vi "Teleop.vi"(10 "Match Info":T1={"Autonomous Elapsed Seconds"=0.0, "TeleOp Elapsed Seconds"=0.0, "Disabled Elapsed Seconds"=0.0, "Visited Autonomous"=FALSE, "Visited TeleOp"=FALSE, "Visited Disabled"=FALSE, "Autonomous Settings"={"Autonomous Style"=enum."Independent", "VI Refnum"=refnum}}, 11 "Call Context":T2) -> ()   [LabVIEW 2015]
doc: "This VI is called for each TeleOp packet received from the DS where the robot is not disabled. It is often used to read from the joysticks and update I/O or to update setpoints for timed control loops. It should complete and return within 20 milliseconds or it may miss DS packets."
uses:
  <vilib>/Rock Robotics/WPI/DriverStation/WPI_DriverStationDerivedRobotMode.ctl
  <vilib>/Rock Robotics/WPI/DriverStation/WPI_DriverStationMatch Info.ctl
  <vilib>/Rock Robotics/WPI/Utilities/WPI_GetSetVariantRefNum.vi
  <vilib>/Rock Robotics/Network Tables/NT Write Boolean Array.vi
  <vilib>/Rock Robotics/Network Tables/NT Write Numeric Array.vi
  <vilib>/Rock Robotics/Network Tables/NT Read Boolean.vi
  <vilib>/Rock Robotics/Network Tables/NT Read Number.vi
  Robot Global Data.vi
  <vilib>/Rock Robotics/Network Tables/NT Write Boolean.vi
panel:
  out "Sample Slider 0":dbl(slide) scale=0.0..5.0
  out "Sample Boolean 1":bool
  out "Sample Boolean 0":bool
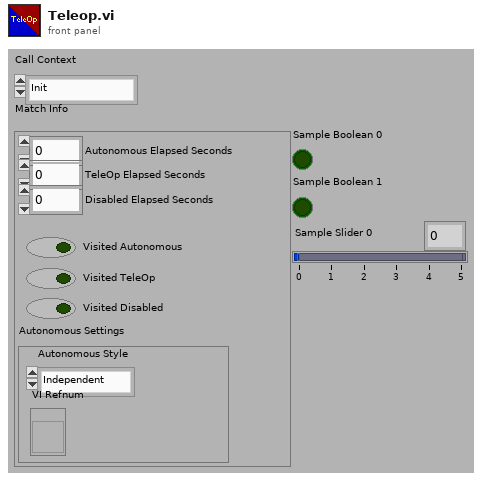
[diagram p1: front panel]
types:
  T1 = typedef "WPI_DriverStationMatch Info.ctl" = cluster{"Autonomous Elapsed Seconds":dbl, "TeleOp Elapsed Seconds":dbl, "Disabled Elapsed Seconds":dbl, "Visited Autonomous":bool, "Visited TeleOp":bool, "Visited Disabled":bool, "Autonomous Settings":cluster{"Autonomous Style":enum16{"Iterative", "Independent"}, "VI Refnum":refnum<vi>}}
  T2 = typedef "WPI_DriverStationDerivedRobotMode.ctl" = enum16{"Init", "Execute", "Stop"}
  T3 = typedef "WPI_RobotDriveDevRef.ctl" = cluster{"DevStatus":errorcluster, "Motors[]":T4[], "Square Inputs":bool, "Max Output":dbl}
  T4 = typedef "WPI_MotorControlDeviceRef.ctl" = cluster{"DeviceStatus":errorcluster, "Type":T5, "PWM":cluster{"PWM Channel":T6, "DeadBand":T7}, "CAN":cluster{"Device Number":u8, "Control Mode":T8, "Semaphore":T9, "Max Vout":dbl, "TalonSRX Control Mode":T10}, "Invert":bool}
  T5 = typedef "WPI_MotorControlType.ctl" = enum16{"PWM", "CAN", "CANTalonSRX"}
  T6 = typedef "FPGA_DIOPWMChannel.ctl" = enum8{"PWM 0", "PWM 1", "PWM 2", "PWM 3", "PWM 4", "PWM 5", "PWM 6", "PWM 7", "PWM 8", "PWM 9", "PWM MXP 0", "PWM MXP 1", "PWM MXP 2", "PWM MXP 3", "PWM MXP 4", "PWM MXP 5", "PWM MXP 6", "PWM MXP 7", "PWM MXP 8", "PWM MXP 9", "Invalid"}
  T7 = typedef "WPI_PWMDeadband.ctl" = cluster{"Name":string, "maxPositivePwm":i32, "minPositivePwm":i32, "centerPwm":i32, "maxNegativePwm":i32, "minNegativePwm":i32, "angularRange":u16}
  T8 = typedef "WPI_CANJaguar_ControlMode.ctl" = enum8{"Percent VBus", "Current", "Speed", "Position", "Voltage"}
  T9 = typedef "Semaphore RefNum" = refnum<k1>
  T10 = typedef "WPI_CANTalonSRX_APIControlMode.ctl" = enum8{"Percent VBus", "Speed", "Position", "Slave", "Unchanged / Invalid", "Voltage Compensation", "Current", "Motion Profile"}
  T11 = typedef "WPI_JoystickDevRef.ctl" = cluster{"Device":T12}
  T12 = typedef "WPI_JoystickDeviceEnum.ctl" = enum16{"USB 0", "USB 1", "USB 2", "USB 3", "USB 4", "USB 5"}
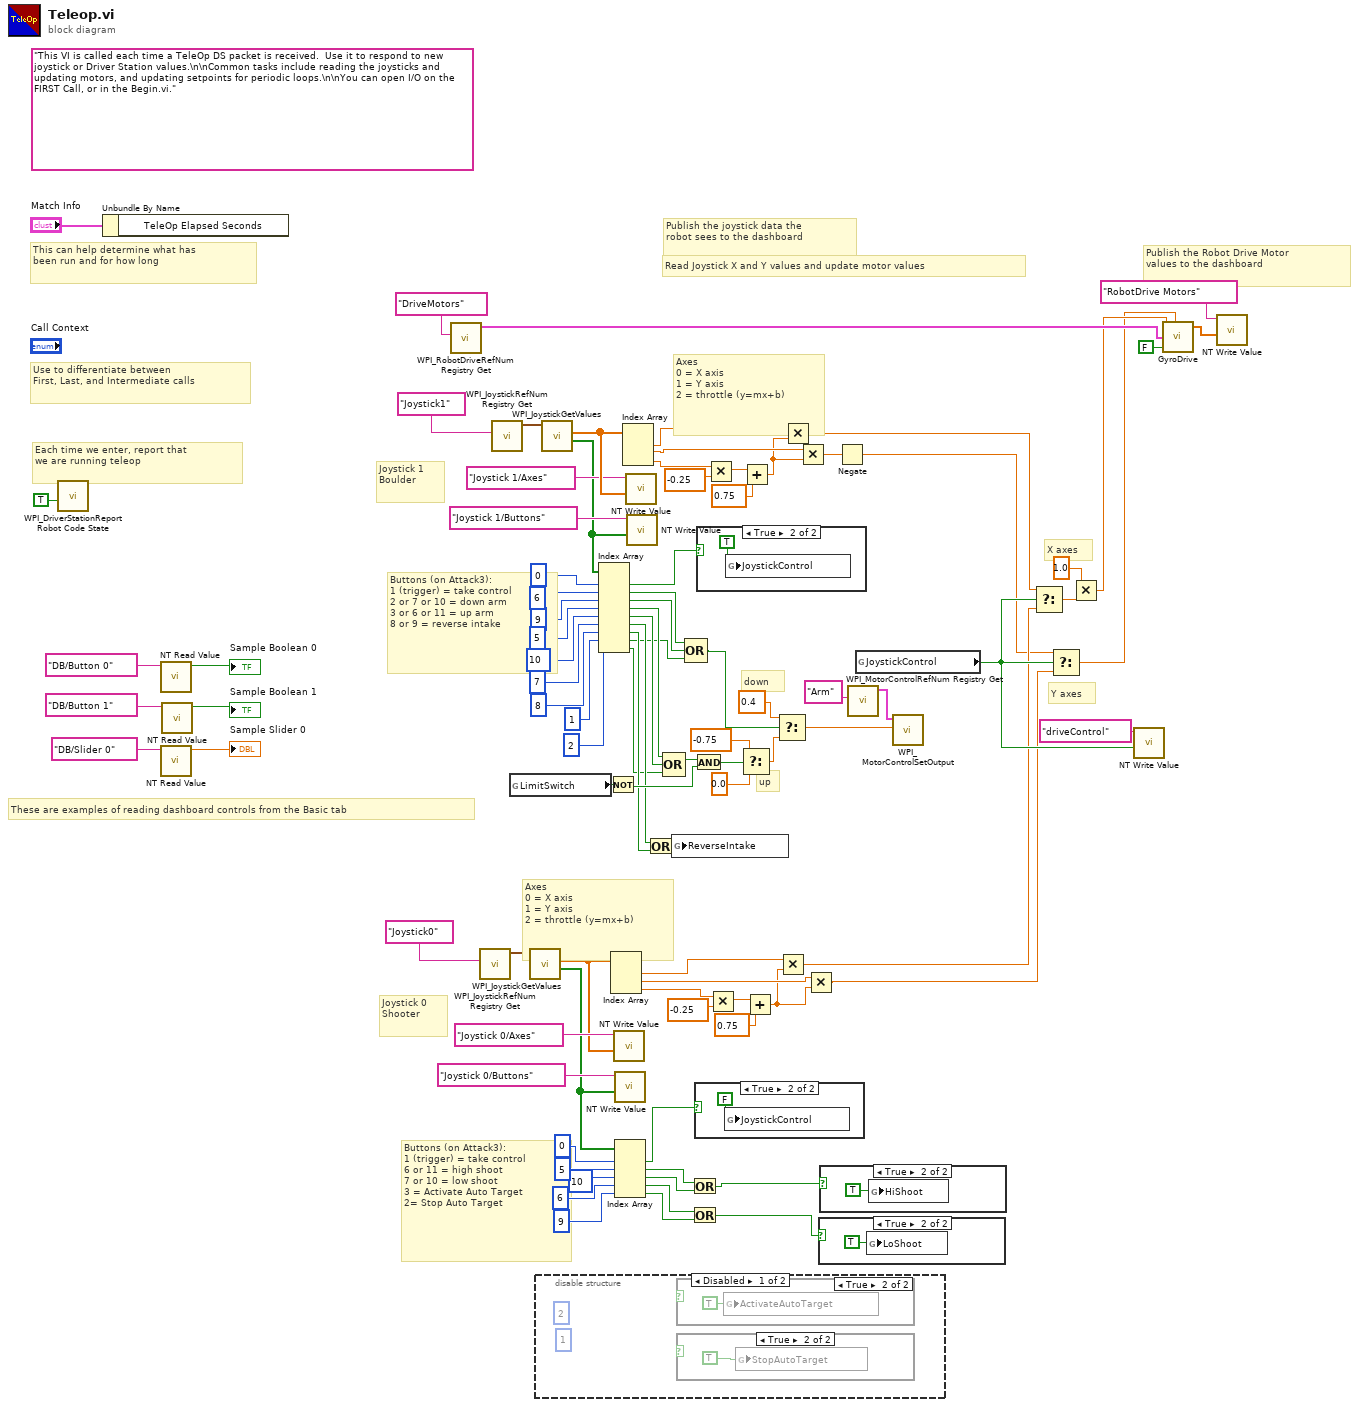
[diagram p0: block diagram]
diagram:
  (unwired) "This VI is called each time a TeleOp DS packet is received.  Use it to respond to new joystick or Driver Station values.\n\nCommon tasks include reading the joysticks and updating motors, and updating setpoints for periodic loops.\n\nYou can open I/O on the FIRST Call, or in the Begin.vi."
  # "up"
  # "down"
  # "Buttons (on Attack3):\n1 (trigger) = take control\n6 or 11 = high shoot\n7 or 10 = low shoot\n3 = Activate Auto Target\n2= Stop Auto Target"
  # "Buttons (on Attack3):\n1 (trigger) = take control\n2 or 7 or 10 = down arm\n3 or 6 or 11 = up arm\n8 or 9 = reverse intake"
  # "Axes\n0 = X axis\n1 = Y axis\n2 = throttle (y=mx+b)"
  # "Axes\n0 = X axis\n1 = Y axis\n2 = throttle (y=mx+b)"
  # "Y axes"
  # "X axes"
  # "Joystick 1\nBoulder"
  # "Joystick 0\nShooter"
  # "These are examples of reading dashboard controls from the Basic tab"
  # "Publish the Robot Drive Motor\nvalues to the dashboard"
  # "Publish the joystick data the\nrobot sees to the dashboard"
  # "Each time we enter, report that\nwe are running teleop"
  # "Use to differentiate between\nFirst, Last, and Intermediate calls"
  # "This can help determine what has\nbeen run and for how long"
  # "Read Joystick X and Y values and update motor values"
  n1 = call <vilib>:"WPI_DriverStationReport Robot Code State.vi"("TeleOp"=TRUE ("Autonomous")) -> ()  [unwired: 10 in, 1 out]
  n2 = Unbundle By Name("Match Info") -> ()  [unwired: 1 out]
  n3 = call-poly <vilib>:"NT Read Value.vi"("Name"="DB/Button 0" ("refnum name")) -> ("Boolean"=→"Sample Boolean 0":bool)  [unwired: 9 in, 1 out]
  n4 = call-poly <vilib>:"NT Read Value.vi"("Name"="DB/Slider 0" ("refnum name")) -> ("Numeric"=→"Sample Slider 0":dbl)  [unwired: 9 in, 1 out]
  n5 = call-poly <vilib>:"NT Read Value.vi"("Name"="DB/Button 1" ("refnum name")) -> ("Boolean"=→"Sample Boolean 1":bool)  [unwired: 9 in, 1 out]
  n6 = call <vilib>:"WPI_RobotDriveRefNum Registry Get.vi"("refnum name"="DriveMotors") -> ("RobotDriveDevRef"=w5:T3)  [unwired: 1 in, 9 out]
  n7 = call <vilib>:"WPI_JoystickRefNum Registry Get.vi"("refnum name"="Joystick0") -> ("JoystickDevRef"=w90:T11)  [unwired: 1 in, 9 out]
  n8 = call <vilib>:"WPI_JoystickRefNum Registry Get.vi"("refnum name"="Joystick1") -> ("JoystickDevRef"=w75:T11)  [unwired: 1 in, 9 out]
  n9 = global read "Robot Global Data.vi" "LimitSwitch"() -> (w32:bool)
  n10 = call <vilib>:"WPI_JoystickGetValues.vi"("JoystickDevRef"=w90) -> ("Buttons"=w69:bool[], "Axes"=w86:dbl[])  [unwired: 6 in, 3 out]
  n11 = disable-structure shown="Disabled" {
    frame Disabled {
      (unwired) 1 ("index")
      (unwired) 2 ("index")
      n12 = case shown="True" {
        selector: _ -> [_ _]
        frame False {
        }
        frame True {
          n13 = global write "Robot Global Data.vi" "ActivateAutoTarget"(TRUE) -> ()
        }
      }
      n14 = case shown="True" {
        selector: _ -> [_ _]
        frame False {
        }
        frame True {
          n15 = global write "Robot Global Data.vi" "StopAutoTarget"(TRUE) -> ()
        }
      }
    }
    frame Enabled {
    }
  }
  n16 = call <vilib>:"WPI_JoystickGetValues.vi"("JoystickDevRef"=w75) -> ("Buttons"=w71:bool[], "Axes"=w78:dbl[])  [unwired: 6 in, 3 out]
  n17 = Index Array(array=w71, index #1=0 ("index"), index #2=6 ("index"), index #3=9 ("index"), index #4=5 ("index"), index #5=10 ("index"), index #6=7 ("index"), index #7=8 ("index"), index #8=1 ("index"), index #9=2 ("index")) -> (element #1=w70:bool, element #2=w10:bool, element #3=w9:bool, element #4=w34:bool, element #5=w33:bool, element #6=w18:bool, element #7=w17:bool, element #8=w8:bool, element #9=w7:bool)
  n18 = Not(x=w32) -> (.not. x?=w30:bool)
  n19 = Index Array(array=w86) -> (element #1=w64:dbl, element #2=w62:dbl, element #3=w66:dbl)  [unwired: 3 in]
  n20 = call-poly <vilib>:"NT Write Value.vi"("Numeric Array"=w86, "Name"="Joystick 0/Axes") -> ()  [unwired: 9 in, 1 out]
  n21 = call-poly <vilib>:"NT Write Value.vi"("Boolean Array"=w69, "Name"="Joystick 0/Buttons") -> ()  [unwired: 9 in, 1 out]
  n22 = Index Array(array=w69, index #1=0 ("index"), index #2=5 ("index"), index #3=10 ("index"), index #4=6 ("index"), index #5=9 ("index")) -> (element #1=w42:bool, element #2=w39:bool, element #3=w38:bool, element #4=w28:bool, element #5=w27:bool)
  n23 = Index Array(array=w78) -> (element #1=w52:dbl, element #2=w54:dbl, element #3=w55:dbl)  [unwired: 3 in]
  n24 = call-poly <vilib>:"NT Write Value.vi"("Numeric Array"=w78, "Name"="Joystick 1/Axes") -> ()  [unwired: 9 in, 1 out]
  n25 = call-poly <vilib>:"NT Write Value.vi"("Boolean Array"=w71, "Name"="Joystick 1/Buttons") -> ()  [unwired: 9 in, 1 out]
  n26 = Or(x=w18, y=w17) -> (x .or. y?=w19:bool)
  n27 = Compound Arithmetic op=OR(w34, w33, w7) -> (w31:bool)
  n28 = global write "Robot Global Data.vi" "ReverseIntake"(w19) -> ()
  n29 = Compound Arithmetic op=OR(w10, w9, w8) -> (w11:bool)
  n30 = Or(x=w39, y=w38) -> (x .or. y?=w22:bool)
  n31 = Or(x=w28, y=w27) -> (x .or. y?=w21:bool)
  n32 = And(x=w31, y=w30) -> (x .and. y?=w29:bool)
  n33 = case shown="True" w42 {
    frame False {
    }
    frame True {
      n34 = global write "Robot Global Data.vi" "JoystickControl"(FALSE) -> ()
    }
  }
  n35 = case shown="True" w70 {
    frame False {
    }
    frame True {
      n36 = global write "Robot Global Data.vi" "JoystickControl"(TRUE) -> ()
    }
  }
  n37 = Multiply(x=w55, y=-0.25) -> (x*y=w57:dbl)
  n38 = Multiply(x=w66, y=-0.25) -> (x*y=w61:dbl)
  n39 = Select(t=-0.75, s=w29, f=0.0) -> (s? t:f=w44:dbl)
  n40 = Add(x=w57, y=0.75) -> (x+y=w53:dbl)
  n41 = Add(x=w61, y=0.75) -> (x+y=w59:dbl)
  n42 = Select(t=0.4, s=w11, f=w44) -> (s? t:f=w43:dbl)
  n43 = Multiply(x=w64, y=w59) -> (x*y=w63:dbl)
  n44 = Multiply(x=w52, y=w53) -> (x*y=w51:dbl)
  n45 = Multiply(x=w54, y=w53) -> (x*y=w49:dbl)
  n46 = Multiply(x=w62, y=w59) -> (x*y=w50:dbl)
  n47 = case shown="True" w21 {
    frame False {
    }
    frame True {
      n48 = global write "Robot Global Data.vi" "LoShoot"(TRUE) -> ()
    }
  }
  n49 = case shown="True" w22 {
    frame False {
    }
    frame True {
      n50 = global write "Robot Global Data.vi" "HiShoot"(TRUE) -> ()
    }
  }
  n51 = Negate(x=w49) -> (-x=w48:dbl)
  n52 = call <vilib>:"WPI_MotorControlRefNum Registry Get.vi"("refnum name"="Arm") -> ("MotorControlDevRef"=w16:T4)  [unwired: 9 in, 1 out]
  n53 = global read "Robot Global Data.vi" "JoystickControl"() -> (w68:bool)
  n54 = call <vilib>:"WPI_MotorControlSetOutput.vi"("Output"=w43, "MotorControlDevRef"=w16) -> ()  [unwired: 7 in, 3 out]
  n55 = Select(t=w51, s=w68, f=w63) -> (s? t:f=w73:dbl)
  n56 = Select(t=w48, s=w68, f=w50) -> (s? t:f=w2:dbl)
  n57 = Multiply(x=1.0, y=w73) -> (x*y=w3:dbl)
  n58 = call-poly <vilib>:"NT Write Value.vi"("Boolean"=w68, "Name"="driveControl") -> ()  [unwired: 9 in, 1 out]
  n59 = call "GyroDrive.vi"("X axis value"=w3, "Y axis value"=w2, "RobotDriveDevRef_In"=w5, "Use gyro"=FALSE) -> ("Motor Values"=w4:dbl[])  [unwired: 1 in, 2 out]
  n60 = call-poly <vilib>:"NT Write Value.vi"("Numeric Array"=w4, "Name"="RobotDrive Motors") -> ()  [unwired: 9 in, 1 out]
